vi "1L05-tb1D-Rech-y_de_F(y).vi"(1 "F(y)":dbl, 2 "F(x)":dbl[](array[numeric]), 3 "x":dbl[](array[numeric])) -> (0 "y interpolé":dbl)   [LabVIEW 2010, in "lv_01.lvlib"]
doc: "Soit en entrée les tableaux 1D x et F(x), le VI retourne la valeur y pour F(y) en entrée. \nTraitement par interpolation même si la valeur de F(y) n'a pas de correspondance dans le tableau F(x)"
uses:
  lv_01.lvlib
panel:
  # "Identifier / Utiliser"
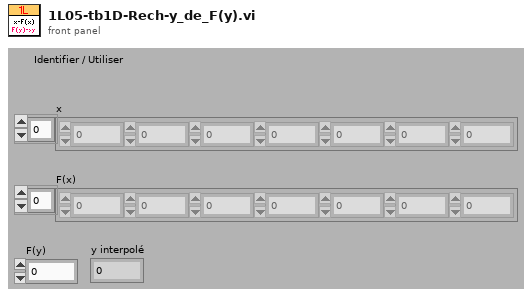
[diagram p1: front panel]
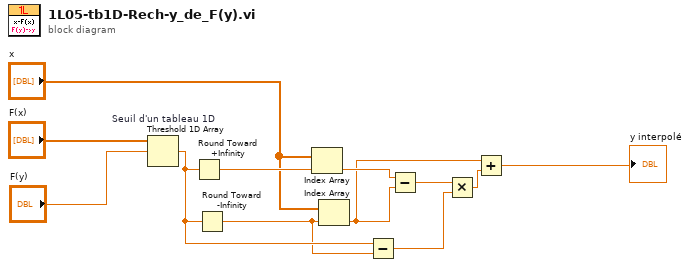
[diagram p0: block diagram]
diagram:
  n1 = Threshold 1D Array "Seuil d'un tableau 1D"(2:"F(y)", 3:"F(x)") -> (0:w3:dbl)  [unwired: 1 in]
  n2 = Round Toward +Infinity(x=w3) -> (ceil(x): smallest int >= x=w10:dbl)
  n3 = Round Toward -Infinity(1:w3) -> (0:w2:dbl)
  n4 = Index Array(array="x", index=w10) -> (element=w8:dbl)
  n5 = Index Array(array="x", index=w2) -> (element=w5:dbl)
  n6 = Subtract(x=w3, y=w2) -> (x-y=w1:dbl)
  n7 = Subtract(x=w8, y=w5) -> (x-y=w7:dbl)
  n8 = Multiply(x=w7, y=w1) -> (x*y=w6:dbl)
  n9 = Add(x=w5, y=w6) -> (x+y=→"y interpolé":dbl)
